vi "GenerateMarvelSeriesMap.vi"(7 "key set":set{cluster{"clz.key":i32, "marvel.key":i32}}(c389), 8 "error in (no error)":errorcluster, 11 "map 2":map{i32, string}(c390)) -> (0 "error out":errorcluster, 3 "map":map{i32, string}(c390))   [LabVIEW 2024]
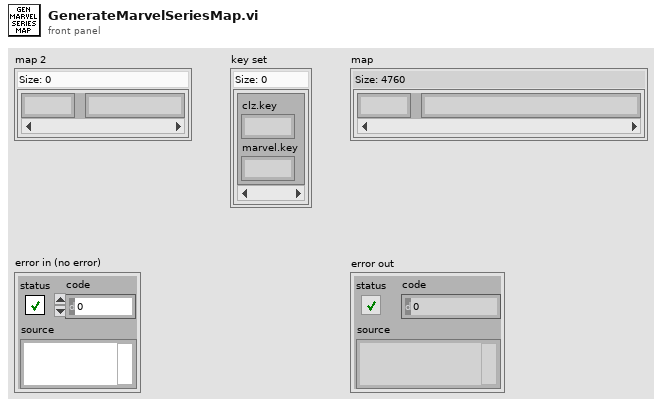
[diagram p1: front panel]
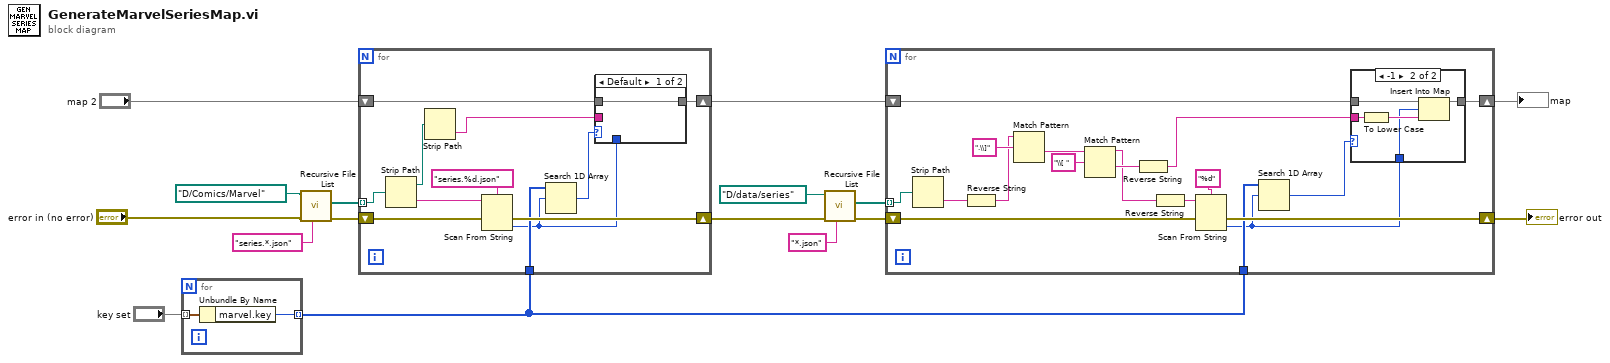
[diagram p0: block diagram]
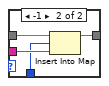
[diagram p2: hidden frame]
diagram:
  n1 = for {
    tunnel: "key set" -> [w18] mode=indexing
    tunnel: [w17] -> w1 mode=indexing
    n2 = Unbundle By Name(w18) -> ("marvel.key"=w17:i32)
  }
  n3 = call <vilib>:"Recursive File List.vi"("pattern"="series.*.json", "error in (no error)"="error in (no error)", "Folder Path"=path "D:/Comics/Marvel") -> ("error out"=w14:errorcluster, "All Files in Dir"=w13:path[])  [unwired: 4 in, 3 out]
  n4 = for {
    tunnel: w13 -> [w30] mode=indexing
    shift-right: [w26] -> w7
    shift-left: w14 -> [w27]
    shift-right: [w24] -> w6
    shift-left: "map 2" -> [w25]
    tunnel: w1 -> [w21]
    n5 = Strip Path(path=w30) -> (stripped path=w29:path, name=w23:string)
    n6 = Strip Path(path=w29) -> (name=w22:string)  [unwired: 1 out]
    n7 = Scan From String(format string="series.%d.json", input string=w23, error in=w27) -> (error out=w26:errorcluster, output 1=w20:i32)  [unwired: 2 in, 2 out]
    n8 = Search 1D Array(1D array=w21, element=w20) -> (index of element=w19:i32)  [unwired: 1 in]
    n9 = case shown="Default" w19 {
      tunnel: w25 -> [w31 w35]
      tunnel: [w31 w34] -> w24
      tunnel: w22 -> [_ w33]
      tunnel: w20 -> [_ w32]
      frame Default {
      }
      frame -1 {
        n10 = Insert Into Map(map in=w35, key=w32, value=w33) -> (map out=w34:map{i32, string})  [unwired: 2 out]
      }
    }
  }
  n11 = call <vilib>:"Recursive File List.vi"("pattern"="*.json", "error in (no error)"=w7, "Folder Path"=path "D:/data/series") -> ("error out"=w10:errorcluster, "All Files in Dir"=w5:path[])  [unwired: 4 in, 3 out]
  n12 = for {
    tunnel: w5 -> [w53] mode=indexing
    shift-right: [w50] -> w3
    shift-left: w10 -> [w51]
    shift-right: [w48] -> w4
    shift-left: w6 -> [w49]
    tunnel: w1 -> [w38]
    n13 = Strip Path(path=w53) -> (name=w46:string)  [unwired: 1 out]
    n14 = Reverse String(1:w46) -> (0:w45:string)
    n15 = Match Pattern(string=w45, regular expression=".\\]") -> (after substring=w43:string)  [unwired: 1 in, 3 out]
    n16 = Match Pattern(string=w43, regular expression="\\[ ") -> (before substring=w39:string, after substring=w40:string)  [unwired: 1 in, 2 out]
    n17 = Reverse String(1:w40) -> (0:w41:string)
    n18 = Reverse String(1:w39) -> (0:w44:string)
    n19 = Scan From String(format string="%d", input string=w44, error in=w51) -> (error out=w50:errorcluster, output 1=w37:i32)  [unwired: 2 in, 2 out]
    n20 = Search 1D Array(1D array=w38, element=w37) -> (index of element=w36:i32)  [unwired: 1 in]
    n21 = case shown="-1" w36 {
      tunnel: w49 -> [w54 w59]
      tunnel: [w54 w58] -> w48
      tunnel: w41 -> [_ w56]
      tunnel: w37 -> [_ w55]
      frame Default {
      }
      frame -1 {
        n22 = To Lower Case(string=w56) -> (all lower case string=w57:string)
        n23 = Insert Into Map(map in=w59, key=w55, value=w57) -> (map out=w58:map{i32, string})  [unwired: 2 out]
      }
    }
  }
  "map" <- w4
  "error out" <- w3
